vi "PH_PPPA_PowerUnit.src DumpRoss.vi"(0 "i ref in":refnum<vi>, 5 "error in (no error)":errorcluster) -> (14 "i ref out":refnum<vi>, 19 "error out":errorcluster)   [LabVIEW 2014, in "PH_PPPA_PowerUnit.lvlib"]
doc: "This is the action VI of the _StateDumpRoss event case. It checks the Device state. Depending on this the following is done:\n\n1 (RR closed): if SM State = \"Open Ross Relais\" and Ignitron.State Device = on, a state change request is send to SM to get \"Load\"\n2 (RR open): if SM State = \"Close Ross Relais\", a state change request is send to SM to get \"Wait for Shot Cmd\""
uses:
  PH_PPPA_PowerUnit.lvlib
  PH_Basics/PH_StatusHandler/PH_StatusHandler.Status.ctl
  PH_Basics/PH_PowerUnit_BaseClass/PH_PowerUnit_BaseClass.SM States.ctl
  PH_Basics/PH_StatusHandler/PH_StatusHandler.lvlib
  PH_Basics/PH_PowerUnit_BaseClass/PH_PowerUnit_BaseClass.lvlib
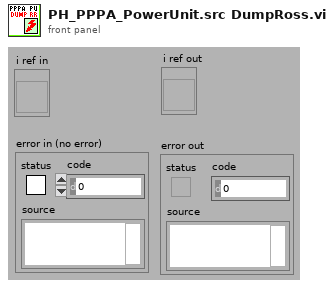
[diagram p1: front panel]
types:
  T1 = typedef "PH_StatusHandler.lvlib/PH_StatusHandler.Status.ctl" = i16
  T2 = typedef "PH_PPPA_PowerUnit.lvlib/PH_PPPA_PowerUnit.i attribute.ctl" = cluster{"GUI Refs":cluster{"Ignitron":refnum<vi>, "Rossrelais":refnum<vi>, "Set Voltage":refnum<vi>, "PSU":refnum<vi>, "EOC":refnum<vi>, "Trigger":refnum<vi>}, "Ignitron":T3, "PSU":T4, "Dump Ross Relais":T5, "Trigger":cluster{"State Device":T1, "linked?":bool}, "Timing Settings":cluster{"Prdc Fast?":bool, "Default Value Periodic Interval":i32, "Mercury on since":dbl, "Warm up Time Mercury [s]":dbl}, "Set Voltage [V]":dbl, "19er Ignitionbox":string}
  T3 = typedef "PH_PP_Common.lvlib/PH_PP_Common.Ignitron Attributes.ctl" = cluster{"State Device":T1, "linked?":bool}
  T4 = typedef "PH_PP_Common.lvlib/PH_PP_Common.PSU Attributes.ctl" = cluster{"lower limit [V]":dbl, "upper limit [V]":dbl, "Voltage set":bool, "State Device":T1, "linked?":bool}
  T5 = typedef "PH_PP_Common.lvlib/PH_PP_Common.Ross Relais Attributes.ctl" = cluster{"State Device":T1, "linked?":bool}
  T6 = typedef "PH_PowerUnit_BaseClass.lvlib/PH_PowerUnit_BaseClass.SM States.ctl" = enum16{".", "Stand by", "Switch PU on", "Configure", "Set Default Voltage", "Set STANDBY", "Set READY", "Wait for Shot Cmd", "Open Dump Rods", "Open Ross Relais", "Close Ross Relais", "Switch PSU on", "Switch PSU off", "Charge", "Switch GD Channel on", "Close Dump Rods", "Rods-TO", "RR-TO", "PSU-TO", "Trigger-TO"}
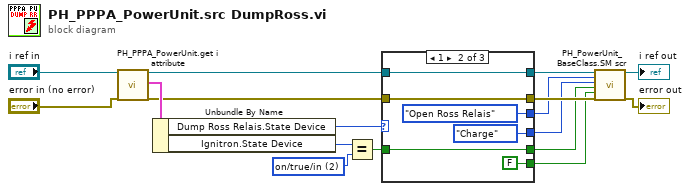
[diagram p0: block diagram]
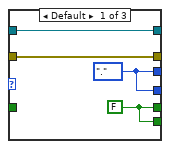
[diagram p2: hidden frame]
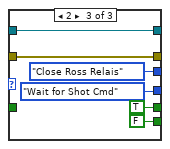
[diagram p3: hidden frame]
diagram:
  w8 = T1 2 items=["no info", "off/false/out", "on/true/in", "Failure", "Alarm", "Status 1", "Status 2", "Status 3"] ("Ignitron.State Device")
  n1 = call "PH_PPPA_PowerUnit.get i attribute.vi"("i ref in"="i ref in", "error in (no error)"="error in (no error)") -> ("i ref out"=w14:refnum<vi>, "i attribute"=w17:T2, "error out"=w13:errorcluster)  [unwired: 15 in]
  n2 = Unbundle By Name(w17) -> ("Dump Ross Relais.State Device"=w11:T1, "Ignitron.State Device"=w10:T1)
  n3 = Equal?(x=w10, y=w8) -> (x = y?=w9:bool)
  n4 = case shown="1" w11 {
    tunnel: w14 -> [w21 w23 w29]
    tunnel: w13 -> [w20 w22 w28]
    tunnel: [w20 w22 w28] -> w12
    tunnel: [w21 w23 w29] -> w6
    tunnel: w9 -> [_ w24 _]
    tunnel: [w18 PH_PowerUnit_BaseClass.SM_States."Open Ross Relais" ("Current SM State (condition)") PH_PowerUnit_BaseClass.SM_States."Close Ross Relais" ("Current SM State (condition)")] -> w4
    tunnel: [w18 PH_PowerUnit_BaseClass.SM_States."Charge" ("Current SM State (condition)") PH_PowerUnit_BaseClass.SM_States."Wait for Shot Cmd" ("Current SM State (condition)")] -> w3
    tunnel: [w19 w24 TRUE] -> w2
    tunnel: [w19 FALSE FALSE] -> w1
    frame Default {
      w19 = FALSE
      w18 = PH_PowerUnit_BaseClass.SM_States."." ("Current SM State (condition)")
    }
    frame 1 {
    }
    frame 2 {
    }
  }
  n5 = call "PH_PowerUnit_BaseClass.SM scr.vi"("VI in"=w6, "Current SM State (condition)"=w4, "Wanted SM State"=w3, "Further change condition"=w2, "PU in use is condition? (true)"=w1, "error in (no error)"=w12) -> ("VI out"=→"i ref out":refnum<vi>, "error out"=→"error out":errorcluster)  [unwired: 12 in]
